vi "CC Script Parse Focus Set Home.vi"(8 "error in (no error)":errorcluster, 9 "To Script?":bool, 10 "Set Home parm in":i32, 11 "DefineObject Parameters":string="Motor=2") -> (0 "error out":errorcluster, 2 "Script Out":string="ObjectName \"RA\":\"123.456\",\"DEC\":\"4546.54\"", 3 "Set Home Parm":i32)   [LabVIEW 2024]
uses:
  <vilib>/regexp/Match Regular Expression.xnode
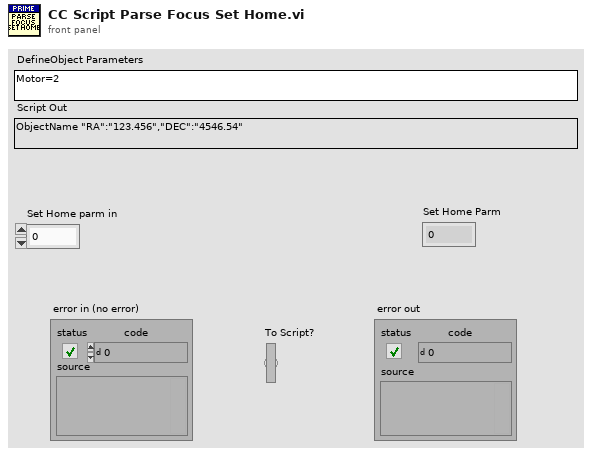
[diagram p1: front panel]
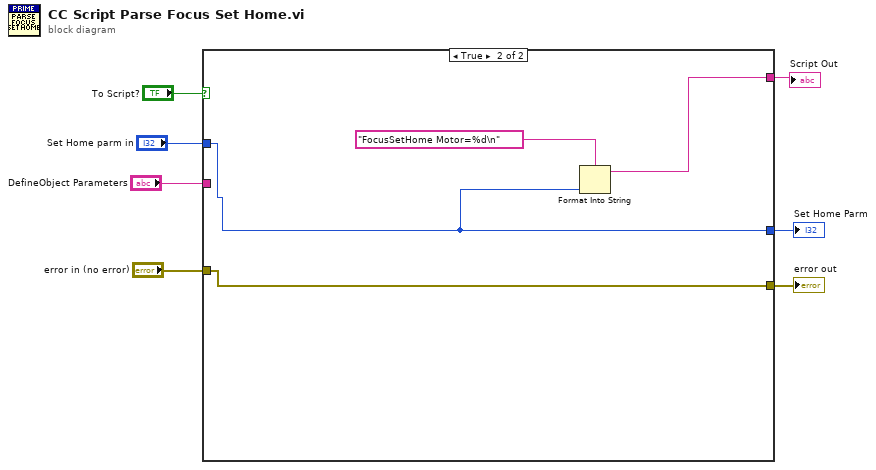
[diagram p0: block diagram]
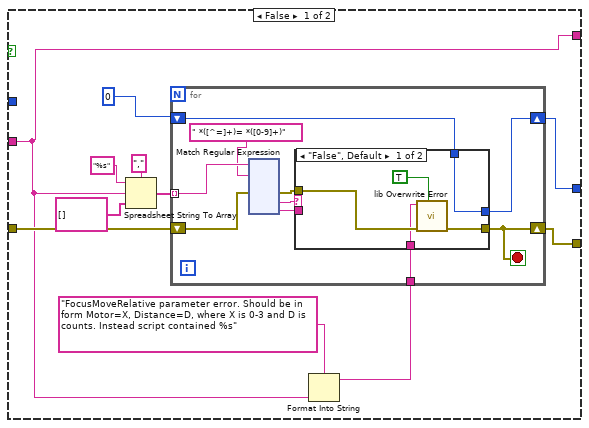
[diagram p2: hidden frame]
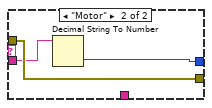
[diagram p3: hidden frame]
diagram:
  n1 = case shown="True" "To Script?" {
    tunnel: [w18 w157] -> w7
    tunnel: "error in (no error)" -> [w17 w158]
    tunnel: [w9 w158] -> w5
    tunnel: "DefineObject Parameters" -> [w12 _]
    tunnel: "Set Home parm in" -> [_ w157]
    tunnel: [w12 w159] -> w2
    frame False {
      n2 = Spreadsheet String To Array(delimiter (Tab)=",", format string="%s", spreadsheet string=w12, array type (2D Dbl)=string[] []) -> (array=w11:string[])
      n3 = Format Into String(format string="FocusMoveRelative parameter error. Should be in form Motor=X, Distance=D, where X is 0-3 and D is counts. Instead script contained %s", w12) -> (resulting string=w10:string)  [unwired: 2 in, 1 out]
      n4 = for {
        shift-right: [w27] -> w18
        shift-left: 0 -> [w28]
        tunnel: w11 -> [w26] mode=indexing
        tunnel: w10 -> [w20]
        shift-right: [w19] -> w9
        shift-left: w17 -> [w22]
        stop <- w19 stop-if-true
        n5 = xnode "Match Regular Expression"("input string"=w26, "regular expression"=" *([^=]+)= *([0-9]+)" ("format string"), "error in"=w22) -> ("error out"=w21:errorcluster, "submatch 1"=w24:string, "submatch 2"=w23:string)  [unwired: 3 in, 4 out]
        n6 = case shown="\"False\", Default" w24 {
          tunnel: w28 -> [w30 _]
          tunnel: [w30 w34] -> w27
          tunnel: w23 -> [_ w35]
          tunnel: w21 -> [w33 w36]
          tunnel: w20 -> [w32 _]
          tunnel: [w31 w36] -> w19
          frame "False", Default {
            n7 = call "lib Overwrite Error.vi"("Force Error?"=TRUE, "error in (no error)"=w33, "Error Message"=w32) -> ("error out"=w31:errorcluster)  [unwired: 8 in]
          }
          frame "Motor" {
            n8 = Decimal String To Number(string=w35) -> (number=w34:i32)  [unwired: 2 in, 1 out]
          }
        }
      }
    }
    frame True {
      n9 = Format Into String(format string="FocusSetHome Motor=%d\n", w157) -> (resulting string=w159:string)  [unwired: 2 in, 1 out]
    }
  }
  "error out" <- w5
  "Set Home Parm" <- w7
  "Script Out" <- w2
